vi "Test Type Selection Prototype.vi"() -> ()   [LabVIEW 2013]
uses:
  Controls/ALTS-2015 Station Cluster.ctl
  Controls/ALTS-2015 LV2GBL Options.ctl
  SLL DAQ Engine/Software/Source Code/Sub VIs/DAQ Engine/Controls/SLL DE List of Digital Inputs.ctl
  SLL DAQ Engine/Software/Source Code/Sub VIs/DAQ Engine/Controls/SLL DE DI Global Options.ctl
panel:
  out "Test Type Selection Successful":bool
  out "TTB":bool
  out "TTA":bool
  in  "stop":bool
  out "error out":errorcluster
  in  "Test Type In":i32
  # "Test Type1: TTA:1, TTB: 0\n\nTest Type2: TTA:0, TTB: 1\n\nTest Type3: TTA:1, TTB: 1\n\nTest Type4: TTA:0, TTB: 0"
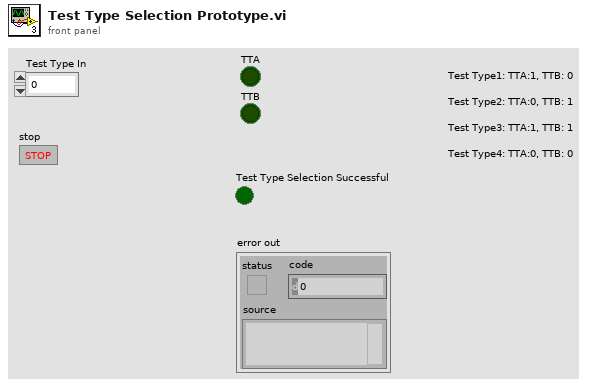
[diagram p1: front panel]
types:
  T1 = typedef "SLL DE List of Digital Inputs.ctl" = enum16{"STATION1_START", "STATION1_STOP", "STATION1_CLAMPED", "STATION1_TC_PASS", "STATION1_TC_FAIL", "STATION1_TTA", "STATION1_TTB", "STATION2_START", "STATION2_STOP", "STATION2_CLAMPED", "STATION2_TC_PASS", "STATION2_TC_FAIL", "STATION2_TTA", "STATION2_TTB", "STATION3_START", "STATION3_STOP", "STATION3_CLAMPED", "STATION3_TC_PASS", "STATION3_TC_FAIL", "STATION3_TTA", "STATION3_TTB", "STATION4_START", "STATION4_STOP", "STATION4_CLAMPED", "STATION4_TC_PASS", "STATION4_TC_FAIL", "STATION4_TTA", "STATION4_TTB"}
  T2 = typedef "ALTS-2015 LV2GBL Options.ctl" = enum16{"Read all", "Write all"}
  T3 = typedef "ALTS-2015 Station Cluster.ctl" = enum16{"Station 1", "Station 2", "Station 3", "Station 4"}
  T4 = typedef "SLL DE DI Global Options.ctl" = enum16{"Init", "Write Line", "Write Array", "Read Line", "Read Array", "Read Full Status", "Write Full Status"}
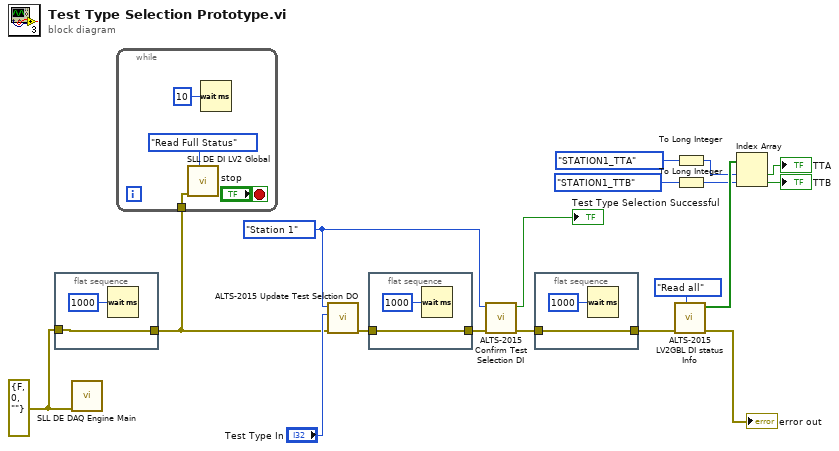
[diagram p0: block diagram]
diagram:
  w17 = ALTS-2015_Station_Cluster."Station 1" ("Station Cluster")
  w9 = errorcluster {"status"=FALSE, "code"=0, "source"=""} ("error in (no error)")
  n1 = flat-sequence {
    tunnel: w9 -> [w19]
    tunnel: [w19] -> w8
    frame #0 {
      n2 = Wait (ms)(milliseconds to wait=u32 1000) -> ()  [unwired: 1 out]
    }
  }
  n3 = call "SLL DE DAQ Engine Main.vi"("error in (no error)"=w9) -> ()  [unwired: 10 in, 1 out]
  n4 = while {
    tunnel: w8 -> [w23]
    stop <- "stop" stop-if-true
    n5 = call "SLL DE DI LV2 Global.vi"("Option"=SLL_DE_DI_Global_Options."Read Full Status", "error in (no error)"=w23) -> ()  [unwired: 6 in, 4 out]
    n6 = Wait (ms)(milliseconds to wait=u32 10) -> ()  [unwired: 1 out]
  }
  n7 = call "ALTS-2015 Update Test Selction DO.vi"("error in"=w8, "Test Type In"="Test Type In", "Station Cluster"=w17) -> ("error out"=w4:errorcluster)  [unwired: 8 in]
  n8 = flat-sequence {
    tunnel: [w25] -> w5
    tunnel: w4 -> [w25]
    frame #0 {
      n9 = Wait (ms)(milliseconds to wait=u32 1000) -> ()  [unwired: 1 out]
    }
  }
  n10 = call "ALTS-2015 Confirm Test Selection DI.vi"("error in"=w5, "Station Cluster"=w17) -> ("error out"=w3:errorcluster, "Test Type Selection Successful"=→"Test Type Selection Successful":bool)  [unwired: 8 in]
  n11 = flat-sequence {
    tunnel: [w27] -> w2
    tunnel: w3 -> [w27]
    frame #0 {
      n12 = Wait (ms)(milliseconds to wait=u32 1000) -> ()  [unwired: 1 out]
    }
  }
  n13 = call "ALTS-2015 LV2GBL DI status Info.vi"("Options"=ALTS-2015_LV2GBL_Options."Read all", "error in"=w2) -> ("error out"=→"error out":errorcluster, "DI Status Out"=w15:bool[])  [unwired: 8 in]
  n14 = To Long Integer(number=SLL_DE_List_of_Digital_Inputs."STATION1_TTA" ("DI Channel Name")) -> (32bit integer=w11:i32)
  n15 = To Long Integer(number=SLL_DE_List_of_Digital_Inputs."STATION1_TTB" ("DI Channel Name")) -> (32bit integer=w12:i32)
  n16 = Index Array(array=w15, index #1=w11, index #2=w12) -> (element #1=→"TTA":bool, element #2=→"TTB":bool)
